vi "Serviceman panel.vi"() -> ()   [LabVIEW 2018]
uses:
  <vilib>/addons/database/Connection.llb/DB Tools Open Connec (Path).vi
  <vilib>/addons/database/NI_Database_API.lvlib
panel:
  in  "Comment":string="Service comment"
  out "SQL query 2":string
  out "SQL query":string
  out "Database Data":i32(listbox)=-1
  out "Traffic light failure":bool
  in  "Repaired":bool
  in  "Arrived":bool
  in  "Logout":bool
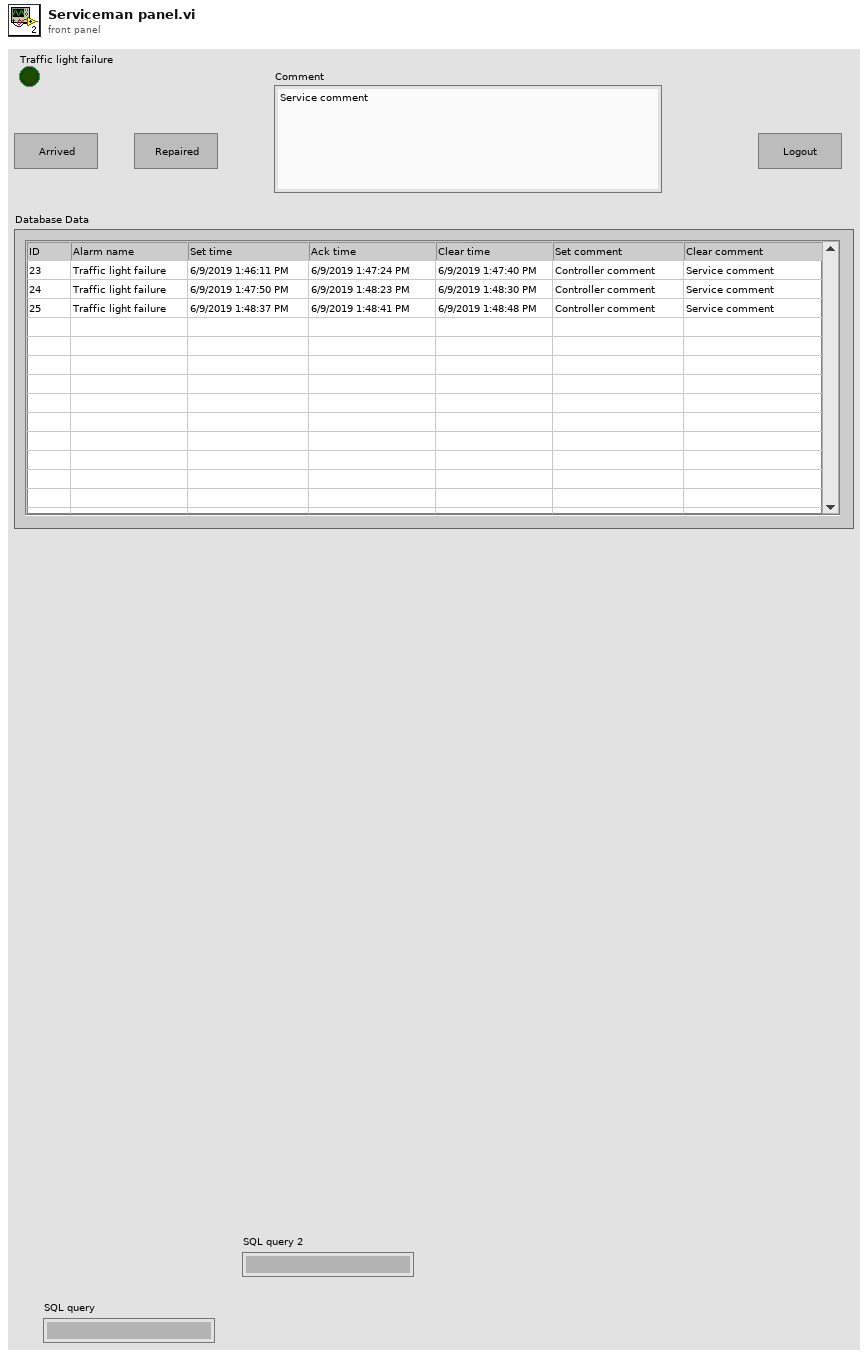
[diagram p1: front panel]
types:
  T1 = typedef "NI_Database_API.lvlib/Conn ObjectReference.ctl" = refnum<k1>
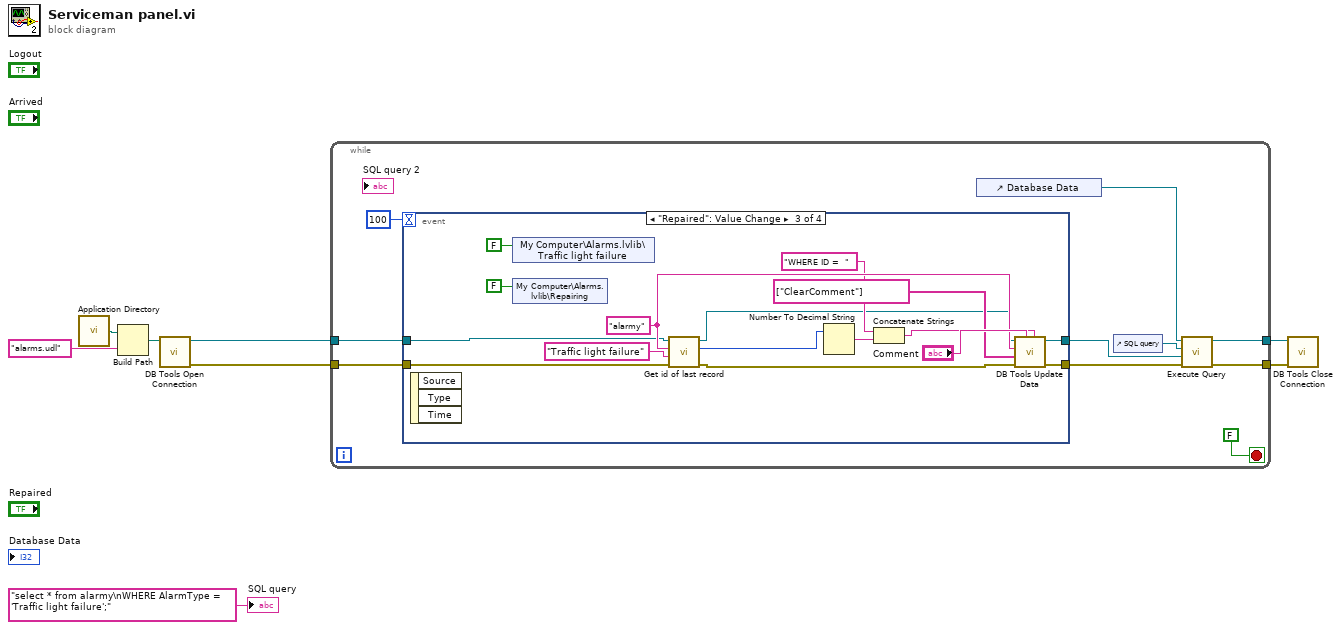
[diagram p0: block diagram]
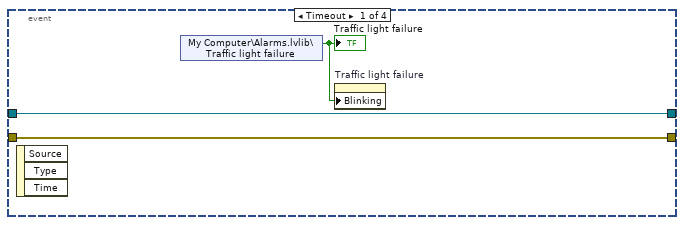
[diagram p2: hidden frame]
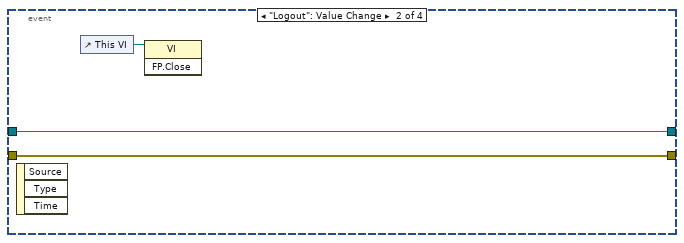
[diagram p3: hidden frame]
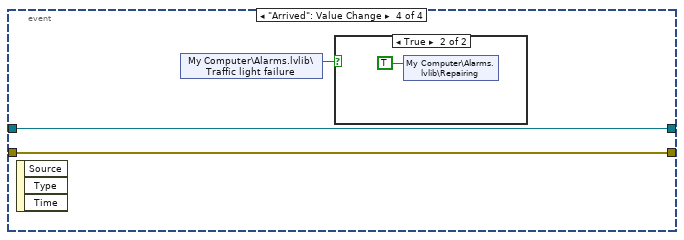
[diagram p4: hidden frame]
diagram:
  n1 = call <vilib>:"Application Directory.vi"() -> ("Application Directory"=w7:path)
  n2 = Build Path(base path=w7, name or relative path="alarms.udl") -> (appended path=w6:path)
  n3 = call-poly <vilib>:"DB Tools Open Connection.vi"("connection information"=w6) -> ("error out"=w1:errorcluster, "connection reference"=w2:T1)  [unwired: 7 in]
  n4 = while {
    tunnel: [w16] -> w4
    tunnel: [w15] -> w3
    tunnel: w2 -> [w13]
    tunnel: w1 -> [w11]
    stop <- FALSE stop-if-true
    n5 = event shown="[2] \"Repaired\": Value Change" {
      selector: _ -> [_ _ _ _]
      dyn-events: _ -> [_ _ _ _]
      timeout: 100 -> [_ _ _ _]
      tunnel: [w20 w23 w25 w42] -> w14
      tunnel: w13 -> [w20 w23 w29 w42]
      tunnel: [w19 w22 w26 w41] -> w12
      tunnel: w11 -> [w19 w22 w28 w41]
      event Timeout {
        n6 = event-data() -> ()  [unwired: 1 in, 3 out]
        n7 = shared-variable "My Computer\\Alarms.lvlib\\Traffic light failure"() -> (w21:bool)  [unwired: 1 in, 1 out]
        "Traffic light failure" <- w21
        n8 = property on="Traffic light failure" class="Bool (strict)"("Blinking"=w21) -> ()  [unwired: 2 in, 2 out]
      }
      event "Logout": Value Change {
        n9 = event-data() -> ()  [unwired: 1 in, 3 out]
        n10 = control-ref of="This VI"() -> (w24:refnum<vi>)
        n11 = invoke class="VI" method="FP.Close"(reference=w24) -> ()  [unwired: 2 in, 3 out]
      }
      event "Repaired": Value Change {
        w37 = "alarmy" ("table")
        n12 = event-data() -> ()  [unwired: 1 in, 3 out]
        n13 = shared-variable "My Computer\\Alarms.lvlib\\Traffic light failure"(FALSE ("Traffic light failure")) -> ()  [unwired: 1 in, 1 out]
        n14 = shared-variable "My Computer\\Alarms.lvlib\\Repairing"(FALSE ("Repairing")) -> ()  [unwired: 1 in, 1 out]
        n15 = call "Get id of last record.vi"("error in (no error)"=w28, "Alarm Type"="Traffic light failure", "table"=w37, "connection reference"=w29) -> ("error out"=w36:errorcluster, "id"=w33:i32, "connection reference 2"=w27:T1)  [unwired: 5 in]
        n16 = Number To Decimal String(number=w33) -> (decimal integer string=w34:string)  [unwired: 1 in]
        n17 = Concatenate Strings("WHERE ID =  " ("SQL query"), w34) -> (w35:string)
        n18 = call <vilib>:"DB Tools Update Data.vi"("condition"=w35, "data"="Comment", "error in (no error)"=w36, "columns"=string[] ["ClearComment"], "table"=w37, "connection reference"=w27) -> ("error out"=w26:errorcluster, "connection reference out"=w25:T1)  [unwired: 4 in]
      }
      event "Arrived": Value Change {
        n19 = event-data() -> ()  [unwired: 1 in, 3 out]
        n20 = shared-variable "My Computer\\Alarms.lvlib\\Traffic light failure"() -> (w43:bool)  [unwired: 1 in, 1 out]
        n21 = case shown="True" w43 {
          frame False {
          }
          frame True {
            n22 = shared-variable "My Computer\\Alarms.lvlib\\Repairing"(TRUE ("Repairing")) -> ()  [unwired: 1 in, 1 out]
          }
        }
      }
    }
    n23 = control-ref of="Database Data"() -> (w9:refnum<vi>)
    n24 = control-ref of="SQL query"() -> (w10:refnum<vi>)
    n25 = call "Execute Query.vi"("error in (no error)"=w12, "connection reference in"=w14, "reference in"=w10, "MulticolumnListbox in"=w9) -> ("error out"=w15:errorcluster, "Refnum out"=w16:T1)  [unwired: 6 in]
  }
  n26 = call <vilib>:"DB Tools Close Connection.vi"("error in (no error)"=w3, "connection reference"=w4) -> ()  [unwired: 5 in, 1 out]
  "SQL query" <- "select * from alarmy\nWHERE AlarmType = 'Traffic light failure';" ("SQL query")
